vi "Loop_TalonSetup (SubVI).vi"(11 "Elbow Setup":T6 {"Feedback Device" items=["None"=-1, "QuadEncoder"=0, "Analog"=2, "Tachometer"=4, "Pulse Width Encoded Position"=8, "Sensor Sum (S0 + S1)"=9, "Sensor Difference (D0 - D1)"=10, "Remote Source 0"=11, "Remote Source 1"=12, "Software Emulated"=15]}) -> (3 "PhoenixMotorControlDevRef":T1)   [LabVIEW 2017]
uses:
  TypeDef/CLUSTER_Talon_Setup.ctl
  System Drivers/Phoenix-LabVIEW/Motor Controller/Controls/CTRE_Phoenix_MotorControl_FeedbackDevice.ctl
  TypeDef/CLUSTER_PID.ctl
  <vilib>/Rock Robotics/WPI/MotorControl/WPI_MotorControlDeviceRef.ctl
  <vilib>/Rock Robotics/WPI/MotorControl/WPI_MotorControlType.ctl
  <vilib>/Rock Robotics/SystemInterfaces/DIO/FPGA_DIOPWMChannel.ctl
  <vilib>/Rock Robotics/WPI/PWM/WPI_PWMDeadband.ctl
  <vilib>/Rock Robotics/SystemInterfaces/DIO/FPGA_DIOChannel.ctl
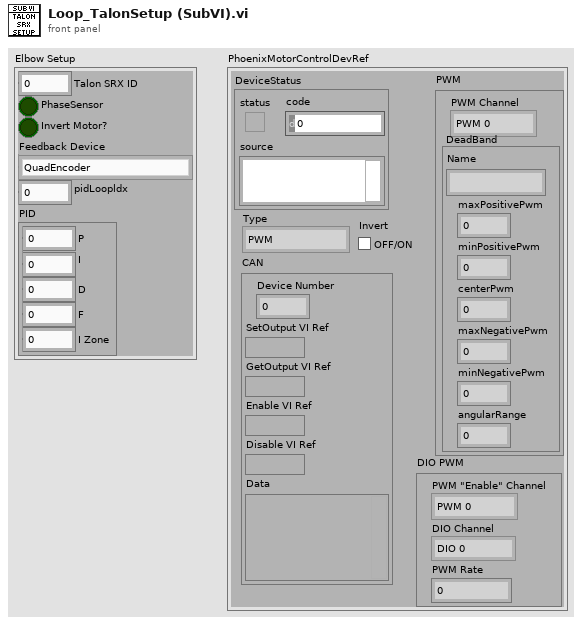
[diagram p1: front panel]
types:
  T1 = typedef "WPI_MotorControlDeviceRef.ctl" = cluster{"DeviceStatus":errorcluster, "Type":T2, "PWM":cluster{"PWM Channel":T3, "DeadBand":T4}, "CAN":cluster{"Device Number":u8, "SetOutput VI Ref":variant, "GetOutput VI Ref":variant, "Enable VI Ref":variant, "Disable VI Ref":variant, "Data":variant}, "Invert":bool, "DIO PWM":cluster{"PWM \"Enable\" Channel":T3, "DIOChannel":T5, "PWM Rate":dbl}}
  T2 = typedef "WPI_MotorControlType.ctl" = enum16{"PWM", "CAN", "DIO PWM"}
  T3 = typedef "FPGA_DIOPWMChannel.ctl" = enum8{"PWM 0", "PWM 1", "PWM 2", "PWM 3", "PWM 4", "PWM 5", "PWM 6", "PWM 7", "PWM 8", "PWM 9", "PWM MXP 0", "PWM MXP 1", "PWM MXP 2", "PWM MXP 3", "PWM MXP 4", "PWM MXP 5", "PWM MXP 6", "PWM MXP 7", "PWM MXP 8", "PWM MXP 9", "Invalid"}
  T4 = typedef "WPI_PWMDeadband.ctl" = cluster{"Name":string, "maxPositivePwm":i32, "minPositivePwm":i32, "centerPwm":i32, "maxNegativePwm":i32, "minNegativePwm":i32, "angularRange":u16}
  T5 = typedef "FPGA_DIOChannel.ctl" = enum8{"DIO 0", "DIO 1", "DIO 2", "DIO 3", "DIO 4", "DIO 5", "DIO 6", "DIO 7", "DIO 8", "DIO 9", "DIO MXP 0", "DIO MXP 1", "DIO MXP 2", "DIO MXP 3", "DIO MXP 4", "DIO MXP 5", "DIO MXP 6", "DIO MXP 7", "DIO MXP 8", "DIO MXP 9", "DIO MXP 10", "DIO MXP 11", "DIO MXP 12", "DIO MXP 13", "DIO MXP 14", "DIO MXP 15", "SPI Port CS1", "SPI Port CS2", "SPI Port CS3", "SPI Port MISO", "SPI Port MOSI", "Invalid"}
  T6 = typedef "CLUSTER_Talon_Setup.ctl" = cluster{"Talon SRX ID":u8, "PhaseSensor":bool, "Invert Motor?":bool, "Phoenix Feedback Select":T7, "pidLoopldx":i32, "PID":T8}
  T7 = typedef "CTRE_Phoenix_MotorControl_FeedbackDevice.ctl" = i8
  T8 = typedef "CLUSTER_PID.ctl" = cluster{"P":dbl, "I":dbl, "D":dbl, "F":dbl, "I Zone":dbl}
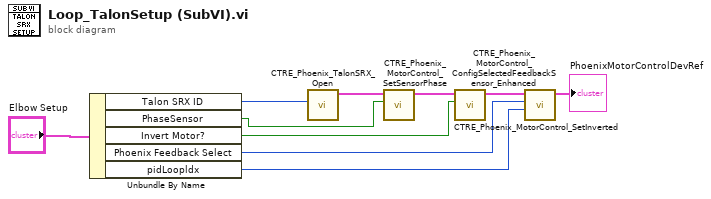
[diagram p0: block diagram]
diagram:
  n1 = Unbundle By Name("Elbow Setup") -> ("Talon SRX ID"=w5:u8, "PhaseSensor"=w4:bool, "Invert Motor?"=w3:bool, "Phoenix Feedback Select"=w2:T7, "pidLoopldx"=w1:i32)
  n2 = call "CTRE_Phoenix_TalonSRX_Open.vi"("Device Number"=w5) -> ("CAN Talon SRX Ref"=w7:T1)  [unwired: 9 in, 1 out]
  n3 = call "CTRE_Phoenix_MotorControl_SetSensorPhase.vi"("PhaseSensor"=w4, "PhoenixMotorControlDevRef"=w7) -> ("PhoenixMotorControlDevRef"=w8:T1)  [unwired: 8 in, 1 out]
  n4 = call "CTRE_Phoenix_MotorControl_SetInverted.vi"("Invert?"=w3, "PhoenixMotorControlDevRef"=w8) -> ("PhoenixMotorControlDevRef"=w9:T1)  [unwired: 8 in, 1 out]
  n5 = call "CTRE_Phoenix_MotorControl_ConfigSelectedFeedbackSensor_Enhanced.vi"("PidLoopIdx"=w1, "Feedback Device"=w2, "PhoenixMotorControlDevRef"=w9) -> ("PhoenixMotorControlDevRef Out"=→"PhoenixMotorControlDevRef":T1)  [unwired: 7 in, 1 out]
